vi "APA_Recognition_sub.vi"(8 "error in (no error)":errorcluster, 11 "IMU_IN[k]":dbl) -> (0 "error out":errorcluster, 2 "Same Sagittal Direction":bool, 3 "Assist Reference":bool)   [LabVIEW 2019]
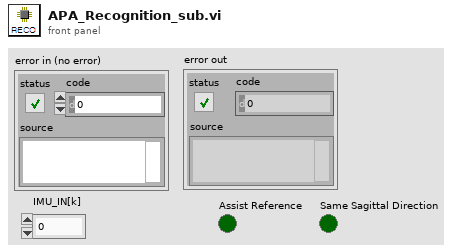
[diagram p1: front panel]
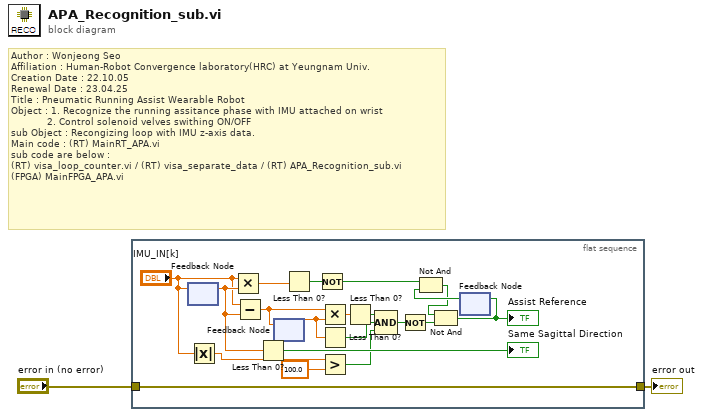
[diagram p0: block diagram]
diagram:
  # "Author : Wonjeong Seo\nAffiliation : Human-Robot Convergence laboratory(HRC) at Yeungnam Univ.\nCreation Date : 22.10.05\nRenewal Date : 23.04.25\nTitle : Pneumatic Running Assist Wearable Robot\nObject : 1. Recognize the running assitance phase with IMU attached on wrist\n            2. Control solenoid velves swithing ON/OFF\nsub Object : Recongizing loop with IMU z-axis data.\nMain code : (RT) MainRT_APA.vi\nsub code are below :\n(RT) visa_loop_counter.vi / (RT) visa_separate_data / (RT) APA_Recognition_sub.vi\n(FPGA) MainFPGA_APA.vi"
  n1 = flat-sequence {
    tunnel: "error in (no error)" -> [w22]
    tunnel: [w22] -> w1
    frame #0 {
      n2 = feedback #1() -> (w20:dbl)  [unwired: 1 in]
      n3 = feedback-in #1("IMU_IN[k]") -> ()
      n4 = Absolute Value(x="IMU_IN[k]") -> (abs(x)=w3:dbl)
      n5 = Multiply(x="IMU_IN[k]", y=w20) -> (x*y=w17:dbl)
      n6 = Subtract(x="IMU_IN[k]", y=w20) -> (x-y=w9:dbl)
      n7 = Less Than 0?(x=w20) -> (x < 0?=→"Same Sagittal Direction":bool)
      n8 = feedback #2() -> (w19:dbl)  [unwired: 1 in]
      n9 = feedback-in #2(w9) -> ()
      n10 = Less Than 0?(x=w17) -> (x < 0?=w14:bool)
      n11 = Not(x=w14) -> (.not. x?=w13:bool)
      n12 = Multiply(x=w9, y=w19) -> (x*y=w18:dbl)
      n13 = Less Than 0?(x=w19) -> (x < 0?=w10:bool)
      n14 = Greater?(x=w3, y=100.0) -> (0:w5:bool)
      n15 = Less Than 0?(x=w18) -> (x < 0?=w11:bool)
      n16 = Compound Arithmetic op=AND(w11, w10, w5) -> (w7:bool)
      n17 = Not(x=w7) -> (.not. x?=w12:bool)
      n18 = feedback #3() -> (w16:bool)  [unwired: 1 in]
      n19 = Not And(1:w16, 2:w13) -> (0:w6:bool)
      n20 = Not And(1:w12, 2:w6) -> (0:w15:bool)
      "Assist Reference" <- w15
      n21 = feedback-in #3(w15) -> ()
    }
  }
  "error out" <- w1
